vi "met_serial_cfg.vi"(8 "error in":errorcluster, 11 "dut serial in":T1={"Baud rate"=9600, "Data bits"=8, "Parity"=0, "Stop bits"=10, "Flow control"=0, "End Mode Read"=enum."None", "End Mode Write"=enum."None", "Term character"=0, "Term enable"=FALSE} {"Flow control" items=["None", "XON/XOFF", "CTS/RTS", "XON/XOFF + CTS/RTS", "DTR/DSR", "XON/XOFF + DTR/DSR"]; "Stop bits" items=["1 bit"=10, "1.5 bits"=15, "2 bits"=20]; "Parity" items=["None", "Odd", "Even", "Mark", "Space"]; "Data bits" items=["5 bits"=5, "6 bits"=6, "7 bits"=7, "8 bits"=8]; "Baud rate" items=["150 Bd"=150, "300 Bd"=300, "600 Bd"=600, "1200 Bd"=1200, "2400 Bd"=2400, "4800 Bd"=4800, "9600 Bd"=9600, "19.2 kBd"=19200, "38.4 kBd"=38400, "57.6 kBd"=57600, "115.2 kBd"=115200]}) -> (0 "error out":errorcluster, 3 "dut serial out":T1={"Baud rate"=9600, "Data bits"=8, "Parity"=0, "Stop bits"=10, "Flow control"=0, "End Mode Read"=enum."None", "End Mode Write"=enum."None", "Term character"=0, "Term enable"=FALSE} {"Flow control" items=["None", "XON/XOFF", "CTS/RTS", "XON/XOFF + CTS/RTS", "DTR/DSR", "XON/XOFF + DTR/DSR"]; "Stop bits" items=["1 bit"=10, "1.5 bits"=15, "2 bits"=20]; "Parity" items=["None", "Odd", "Even", "Mark", "Space"]; "Data bits" items=["5 bits"=5, "6 bits"=6, "7 bits"=7, "8 bits"=8]; "Baud rate" items=["150 Bd"=150, "300 Bd"=300, "600 Bd"=600, "1200 Bd"=1200, "2400 Bd"=2400, "4800 Bd"=4800, "9600 Bd"=9600, "19.2 kBd"=19200, "38.4 kBd"=38400, "57.6 kBd"=57600, "115.2 kBd"=115200]})   [LabVIEW 2020]
uses:
  met_serial_setup.ctl
  varilib/varilib.lvlib
panel:
  in  "btn ok":bool
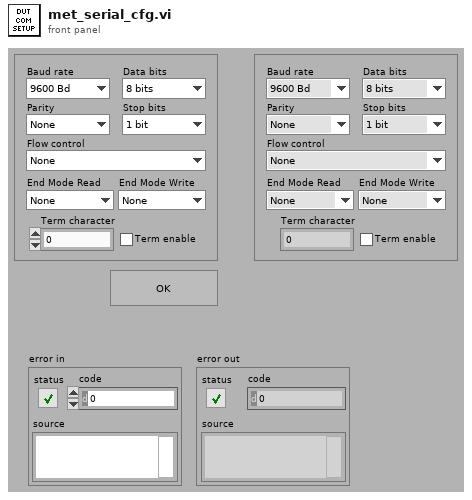
[diagram p1: front panel]
types:
  T1 = typedef "met_serial_setup.ctl" = cluster{"Baud rate":i32, "Data bits":i32, "Parity":i32, "Stop bits":i32, "Flow control":i32, "End Mode Read":enum16{"None", "Last Bit", "TermChar"}, "End Mode Write":enum16{"None", "Last Bit", "TermChar"}, "Term character":u8, "Term enable":bool}
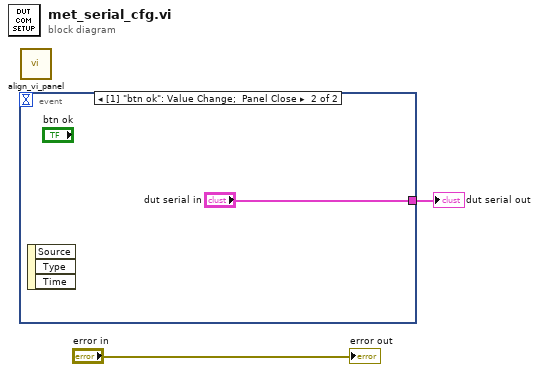
[diagram p0: block diagram]
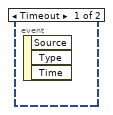
[diagram p2: hidden frame]
diagram:
  n1 = event shown="[1] \"btn ok\": Value Change;  Panel Close" {
    selector: _ -> [_ _]
    dyn-events: _ -> [_ _]
    timeout: _ -> [_ _]
    tunnel: [_ "dut serial in"] -> w1
    event Timeout {
      n2 = event-data() -> ()  [unwired: 1 in, 3 out]
    }
    event "btn ok": Value Change; Panel Close {
      n3 = event-data() -> ()  [unwired: 1 in, 3 out]
    }
  }
  "dut serial out" <- w1
  n4 = call "align_vi_panel.vi"() -> ()  [unwired: 11 in, 1 out]
  "error out" <- "error in"
